vi "ConsignePressionSimu.vi"() -> ()   [LabVIEW 2012]
panel:
  in  "ConsignePressionSimu":dbl
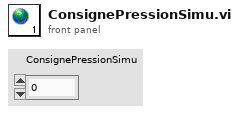
[diagram p1: front panel]
diagram:
